vi "Write Message.vi"(6 "binary?":bool, 8 "error in (no error)":errorcluster, 9 "timeout in ms (-1)":i32=-1, 10 "message":string, 11 "WebSocket Connection in":refnum<class "WebSocket Connection.lvclass">) -> (0 "error out":errorcluster, 3 "WebSocket Connection out":refnum<class "WebSocket Connection.lvclass">)   [LabVIEW 2019, in "WebSocket Server Toolkit.lvlib" / "WebSocket Connection.lvclass"]
uses:
  WebSocket Connection.lvclass
  types/frame_data.ctl
  WebSocket Server Toolkit.lvlib
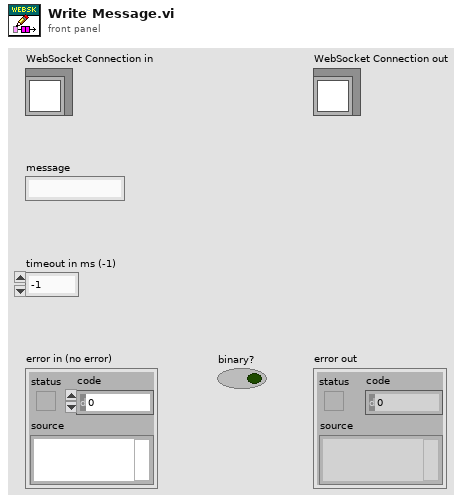
[diagram p1: front panel]
types:
  T1 = typedef "WebSocket Server Toolkit.lvlib/frame_data.ctl" = cluster{"binary?":bool, "frames":string[]}
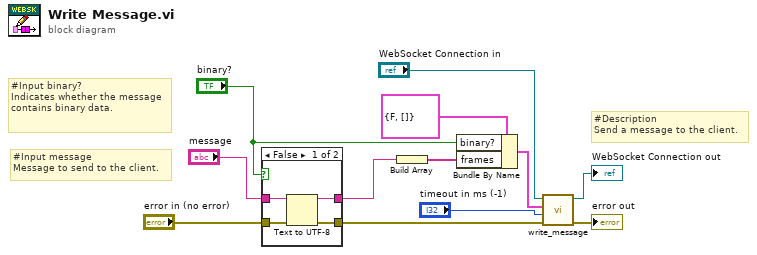
[diagram p0: block diagram]
diagram:
  # "#Input binary?\nIndicates whether the message contains binary data."
  # "#Input message\nMessage to send to the client."
  # "#Description\nSend a message to the client."
  n1 = case shown="False" "binary?" {
    tunnel: "message" -> [w16 w18]
    tunnel: [w15 w18] -> w4
    tunnel: "error in (no error)" -> [w14 w17]
    tunnel: [w13 w17] -> w1
    frame False {
      n2 = Text to UTF-8(8:w14, 11:w16) -> (0:w13:errorcluster, 3:w15:string)  [unwired: 1 in]
    }
    frame True {
    }
  }
  n3 = Build Array(w4) -> (w8:string[])
  n4 = Bundle By Name(cluster=T1 {"binary?"=FALSE, "frames"=[]} ("element"), "binary?"="binary?", "frames"=w8) -> (w7:T1)
  n5 = call-dynamic "write_message.vi"("error in (no error)"=w1, "timeout in ms (-1)"="timeout in ms (-1)", "element"=w7, "WebSocket Connection in"="WebSocket Connection in") -> ("error out"=→"error out":errorcluster, "WebSocket Connection out"=→"WebSocket Connection out":refnum<class "WebSocket Connection.lvclass">)  [unwired: 5 in, 1 out]
